vi "MAUI.Basic.TestLauncher.vi"() -> ()   [LabVIEW 2019, in "MAUI.Basic.lvclass"]
uses:
  MAUI.Basic.lvclass
  <vilib>/JKI/JKI SMO/SMO/Typedefs/SMOState --Enum.ctl
  C:/Program Files (x86)/National Instruments/LabVIEW 2019/vi.lib/JKI/JKI SMO/SMO/SMO.lvclass
  C:/Program Files (x86)/National Instruments/LabVIEW 2019/vi.lib/JKI/JKI SMO/SMO.UI/SMO.UI.lvclass
  C:/Users/patrick/Documents/GitHub/MAUI-Engine/lvsrc/Maui 1.0/SMO.UI.MAUI/MAUI.lvclass
  <vilib>/JKI/JKI SMO/SMO/SMO.lvclass/SMO.ctl
  <vilib>/JKI/JKI SMO/SMO.UI/SMO.UI.lvclass/SMO.UI.ctl
  <vilib>/JKI/JKI SMO/SMO/Private/ReftoDVR--SMO.vi
  <vilib>/JKI/JKI SMO/SMO.UI/SMO.UI.ReftoDVR.vi
  <vilib>/JKI/JKI SMO/SMO/SMO.lvclass
  <vilib>/JKI/JKI SMO/SMO.UI/SMO.UI.lvclass
  Maui 1.0/SMO.UI.MAUI/MAUI.lvclass
panel:
  out "SMO State":T1
  out "error out":errorcluster
  in  "Stop":bool
  # "MAUI SMO Test Launcher"
  # "For instructions on how to use the JKI State Machine Objects, examples and video tutorials, visit:\nhttp://jki.net/state-machine-objects/\n\nJKI State Machine Objects™\nhttp://jki.net/state-machine-objects/\nCopyright (C) 2005-2015, JKI <info@jki.net>\nALL RIGHTS RESERVED"
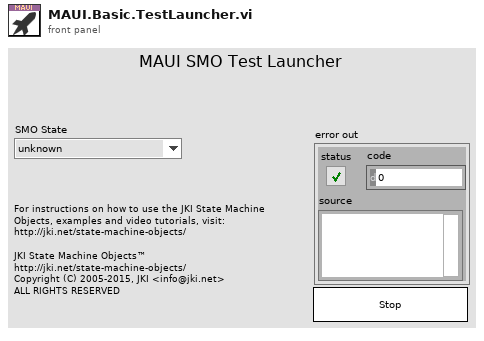
[diagram p1: front panel]
types:
  T1 = typedef "SMO.lvclass/SMOState --Enum.ctl" = enum16{"unknown", "Created", "Started", "Stopped"}
  T2 = typedef "SMO.lvclass/Public Events.ctl" = cluster{"Error":refnum<user-event>, "State":refnum<user-event>, "Reserve State":refnum<user-event>}
  T3 = typedef "SMO.UI.lvclass/PublicEvents--Cluster.ctl" = cluster{"UI Hidden":refnum<user-event>, "UI State":refnum<user-event>}
  T4 = cluster{"Event Registration Refnum":refnum<event-registration>}
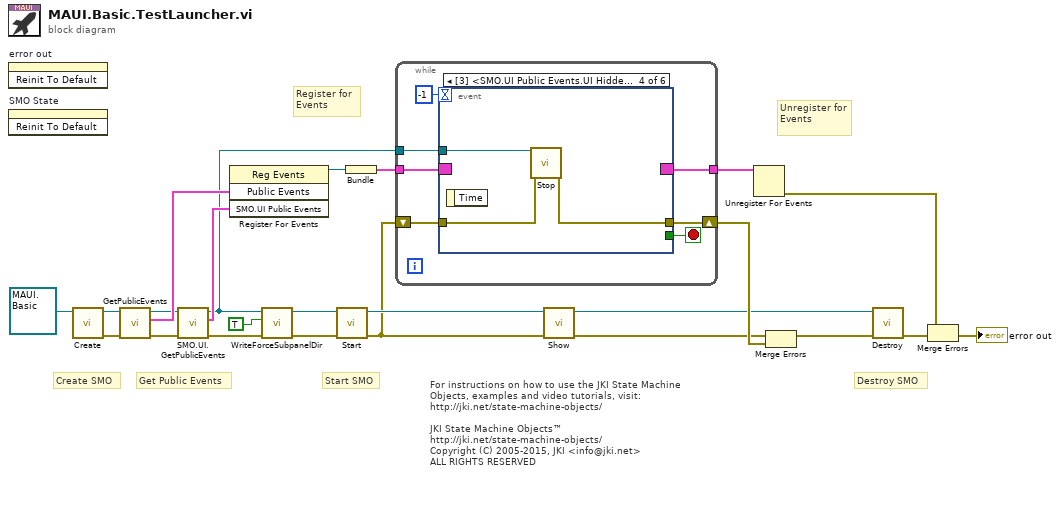
[diagram p0: block diagram]
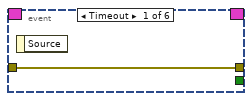
[diagram p2: hidden frame]
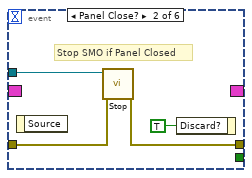
[diagram p3: hidden frame]
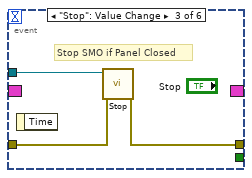
[diagram p4: hidden frame]
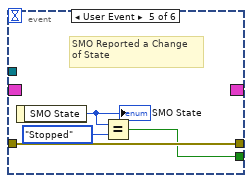
[diagram p5: hidden frame]
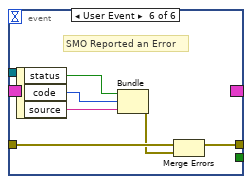
[diagram p6: hidden frame]
diagram:
  # "For instructions on how to use the JKI State Machine Objects, examples and video tutorials, visit:\nhttp://jki.net/state-machine-objects/\n\nJKI State Machine Objects™\nhttp://jki.net/state-machine-objects/\nCopyright (C) 2005-2015, JKI <info@jki.net>\nALL RIGHTS RESERVED"
  # "Get Public Events"
  # "Start SMO"
  # "Destroy SMO"
  # "Create SMO"
  # "Unregister for Events"
  # "Register for Events"
  n1 = invoke on="error out" class="Clust (strict)" method="Reinit To Default"() -> ()  [unwired: 3 in, 3 out]
  n2 = invoke on="SMO State" class="Enum (strict)" method="Reinit To Default"() -> ()  [unwired: 3 in, 3 out]
  n3 = call <vilib>:"Create.vi"("SMO"=refnum<class "MAUI.Basic.lvclass"> refnum ("SMO.Template.lvclass")) -> ("error out"=w15:errorcluster, "SMO out"=w16:refnum<class "MAUI.Basic.lvclass">)  [unwired: 8 in, 1 out]
  n4 = call <vilib>:"GetPublicEvents.vi"("error in (no error)"=w15, "SMO"=w16) -> ("error out"=w2:errorcluster, "Public Events"=w14:T2, "SMO out"=w8:refnum<class "MAUI.Basic.lvclass">)  [unwired: 7 in]
  n5 = call <vilib>:"SMO.UI.GetPublicEvents.vi"("error in (no error)"=w2, "SMO.UI"=w8) -> ("error out"=w1:errorcluster, "SMO.UI Public Events"=w7:T3, "SMO.UI out"=w5:refnum<class "MAUI.Basic.lvclass">)  [unwired: 7 in]
  n6 = register-events(w14, w7) -> (reference out=w13:refnum<event-registration>)  [unwired: 2 in, 1 out]
  n7 = call "WriteForceSubpanelDir.vi"("error in (no error)"=w1, "ForceSubpanelDir?"=TRUE, "SMO.UI.MAUI in"=w5) -> ("error out"=w6:errorcluster, "SMO.UI.MAUI out"=w4:refnum<class "MAUI.Basic.lvclass">)  [unwired: 7 in]
  n8 = call <vilib>:"Start.vi"("error in (no error)"=w6, "SMO"=w4) -> ("error out"=w10:errorcluster, "SMO out"=w12:refnum<class "MAUI.Basic.lvclass">)  [unwired: 8 in]
  n9 = Bundle("Event Registration Refnum"=w13) -> (w23:T4)  [unwired: 1 in]
  n10 = while {
    shift-right: [w30] -> w22
    shift-left: w10 -> [w29]
    tunnel: w23 -> [w28]
    tunnel: [w27] -> w24
    tunnel: w5 -> [w26]
    stop <- w31 stop-if-true
    n11 = event shown="[3] <SMO.UI Public Events.UI Hidden>: User Event" {
      selector: w28 -> [_ _ _ _ _ _]
      dyn-events: [_ _ _ _ _ _] -> w27
      timeout: -1 -> [_ _ _ _ _ _]
      tunnel: [_ _ _ _ w43 _] -> w31
      tunnel: w26 -> [_ w36 w39 w42 _ _]
      tunnel: [w32 w35 w38 w40 w46 w50] -> w30
      tunnel: w29 -> [w32 w34 w37 w41 w46 w48]
      event Timeout {
        n12 = event-data() -> ()  [unwired: 1 in, 1 out]
      }
      event Panel Close? {
        # "Stop SMO if Panel Closed"
        n13 = event-data() -> ()  [unwired: 1 in, 1 out]
        n14 = call <vilib>:"Stop.vi"("error in (no error)"=w34, "SMO"=w36) -> ("error out"=w35:errorcluster)  [unwired: 8 in, 1 out]
        n15 = event-data ("Event Filter Node")("Discard?"=TRUE ("OK")) -> ()  [unwired: 1 in, 1 out]
      }
      event "Stop": Value Change {
        # "Stop SMO if Panel Closed"
        n16 = event-data() -> ()  [unwired: 1 in, 1 out]
        n17 = call <vilib>:"Stop.vi"("error in (no error)"=w37, "SMO"=w39) -> ("error out"=w38:errorcluster)  [unwired: 8 in, 1 out]
      }
      event User Event {
        n18 = event-data() -> ()  [unwired: 1 in, 1 out]
        n19 = call <vilib>:"Stop.vi"("error in (no error)"=w41, "SMO"=w42) -> ("error out"=w40:errorcluster)  [unwired: 8 in, 1 out]
      }
      event User Event {
        # "SMO Reported a Change\nof State"
        n20 = event-data() -> ("SMO State"=w45:T1)  [unwired: 1 in]
        "SMO State" <- w45
        n21 = Equal?(x=w45, y=SMOState_--Enum."Stopped") -> (x = y?=w43:bool)
      }
      event User Event {
        # "SMO Reported an Error"
        n22 = event-data() -> ("status"=w49:bool, "code"=w52:i32, "source"=w51:string)  [unwired: 1 in]
        n23 = Bundle("status"=w49, "code"=w52, "source"=w51) -> (w47:errorcluster)  [unwired: 1 in]
        n24 = Merge Errors(w48, w47) -> (w50:errorcluster)
      }
    }
  }
  n25 = call <vilib>:"Show.vi"("error in (no error)"=w10, "SMO.UI"=w12) -> ("error out"=w9:errorcluster, "SMO.UI out"=w11:refnum<class "MAUI.Basic.lvclass">)  [unwired: 8 in]
  n26 = Unregister For Events(event registration refnum=w24) -> (error out=w21:errorcluster)  [unwired: 1 in]
  n27 = Merge Errors(w9, w22) -> (w17:errorcluster)
  n28 = call <vilib>:"Destroy.vi"("error in (no error)"=w17, "SMO"=w11) -> ("error out"=w19:errorcluster)  [unwired: 9 in]
  n29 = Merge Errors(w21, w19) -> (→"error out":errorcluster)
